vi "kvCanMsgDisplayBox.vi"(1 "Message Data":u8[](array[numeric]), 2 "Message Flags":u32, 3 "Message Id":i32, 4 "Time Stamp":u32) -> (0 "Output String":string)   [LabVIEW 2022 SP3]
doc: "This VI converts the data returned by ncReadNetMult into string format. The Time Format Select input allows the user to chose between absolute timestamps and relative timestamps."
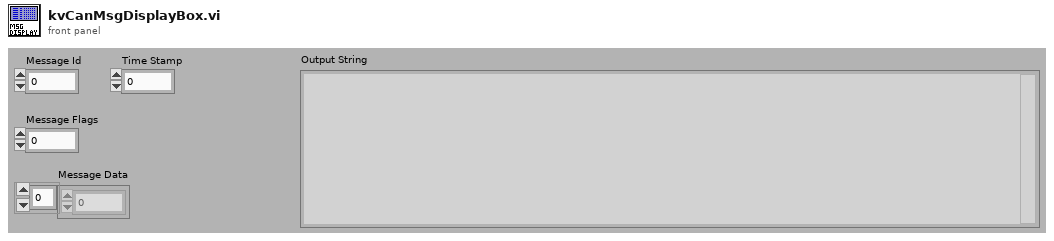
[diagram p1: front panel]
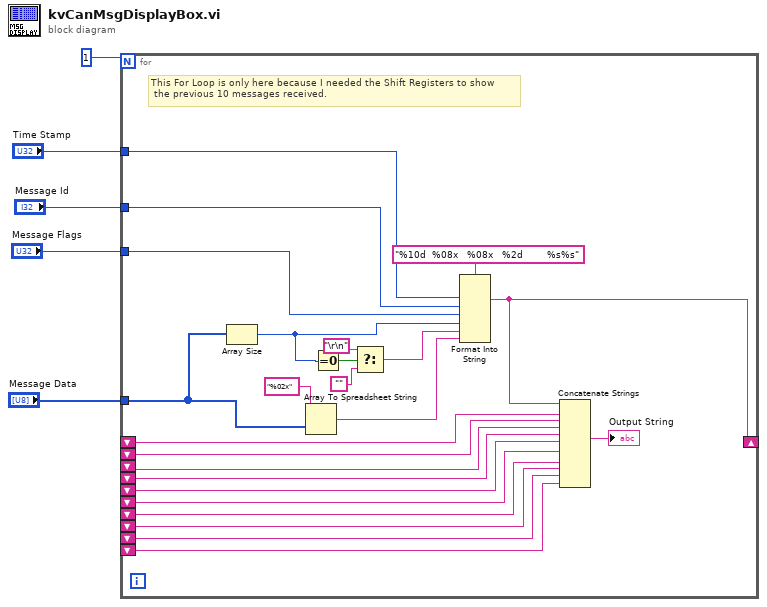
[diagram p0: block diagram]
diagram:
  n1 = for {
    N: 1 -> [_]
    shift-right: [w28] -> _
    shift-left: _ -> [w27]
    shift-left: _ -> [w26]
    shift-left: _ -> [w25]
    shift-left: _ -> [w24]
    shift-left: _ -> [w23]
    shift-left: _ -> [w22]
    shift-left: _ -> [w21]
    shift-left: _ -> [w20]
    shift-left: _ -> [w19]
    shift-left: _ -> [w18]
    tunnel: "Message Id" -> [w15]
    tunnel: "Message Data" -> [w13]
    tunnel: "Time Stamp" -> [w14]
    tunnel: "Message Flags" -> [w6]
    # "This For Loop is only here because I needed the Shift Registers to show\n the previous 10 messages received."
    n2 = Array Size(array=w13) -> (size(s)=w9:i32)
    n3 = Array To Spreadsheet String(array=w13, 3:"%02x" ("format string")) -> (spreadsheet string=w7:string)  [unwired: 1 in]
    n4 = Equal To 0?(x=w9) -> (x = 0?=w12:bool)
    n5 = Select(t="\r\n", s=w12, f="") -> (s? t:f=w8:string)
    n6 = Format Into String(format string="%10d  %08x   %08x   %2d        %s%s", w14, w15, w6, w9, w8, w7) -> (resulting string=w28:string)  [unwired: 2 in, 1 out]
    n7 = Concatenate Strings(w28, w27, w26, w25, w24, w23, w22, w21, w20, w19, w18) -> (→"Output String":string)
  }
